vi "Phi to Gait Lookup v2.vi"(11 "Current Phi":dbl) -> (3 "Current Gait %":dbl)   [LabVIEW 2018]
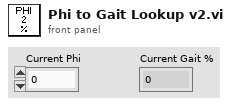
[diagram p1: front panel]
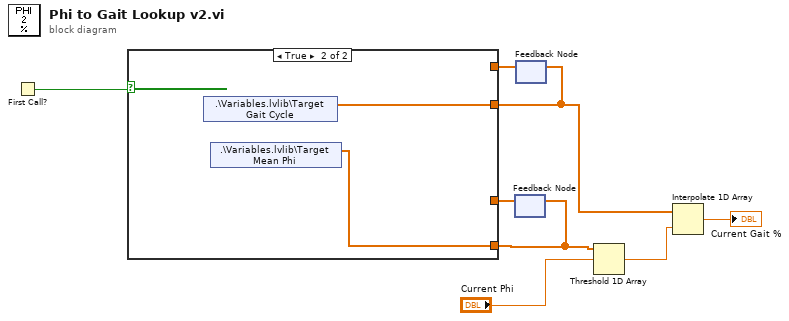
[diagram p0: block diagram]
diagram:
  n1 = First Call?() -> (First Call?: T/F=w5:bool)
  n2 = feedback #1() -> (w1:dbl[])  [unwired: 1 in]
  n3 = feedback #2() -> (w2:dbl[])  [unwired: 1 in]
  n4 = case shown="True" w5 {
    tunnel: [w10 w12] -> w3
    tunnel: [w9 w11] -> w4
    tunnel: w2 -> [w10 _]
    tunnel: w1 -> [w9 _]
    frame False {
    }
    frame True {
      n5 = shared-variable ".\\Variables.lvlib\\Target Gait Cycle"() -> (w12:dbl[])  [unwired: 1 in, 1 out]
      n6 = shared-variable ".\\Variables.lvlib\\Target Mean Phi"() -> (w11:dbl[])  [unwired: 1 in, 1 out]
    }
  }
  n7 = feedback-in #1(w4) -> ()
  n8 = feedback-in #2(w3) -> ()
  n9 = Threshold 1D Array(2:"Current Phi", 3:w4) -> (0:w8:dbl)  [unwired: 1 in]
  n10 = Interpolate 1D Array(1:w8, 2:w3) -> (0:→"Current Gait %":dbl)
